vi "NF LI56xx sub init signal.vi"(7 "Type":string, 8 "error in":errorcluster caption="error in (no error)" {"code" format="%.0x"}, 11 "VISA resource name":refnum<visa-resource-name>) -> (0 "error out":errorcluster {"code" format="%.0x"}, 3 "VISA resource name copy":refnum<visa-resource-name>)   [LabVIEW 2019]
doc: "get input signal related parameters"
panel:
  in  "Measure Cluster":T1
  out "Measure Output Cluster":T2
  in  "Signal Cluster":T3
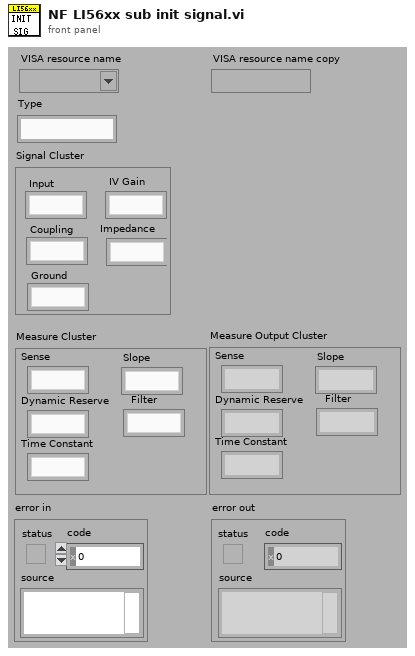
[diagram p1: front panel]
types:
  T1 = cluster{"Sense":string, "Dynamic Reserve":string, "Slope":string, "Filter":string, "Time Constant":string}
  T2 = cluster{"Sense":string, "Dynamic Reserve":string, "Time Constant":string, "Slope":string, "Filter":string}
  T3 = cluster{"Input":string, "Coupling":string, "Ground":string, "IV Gain":string, "Impedance":string}
  T4 = cluster{"input":string, "coupling":string, "ground":string, "IV gain":string, "impedance":string}
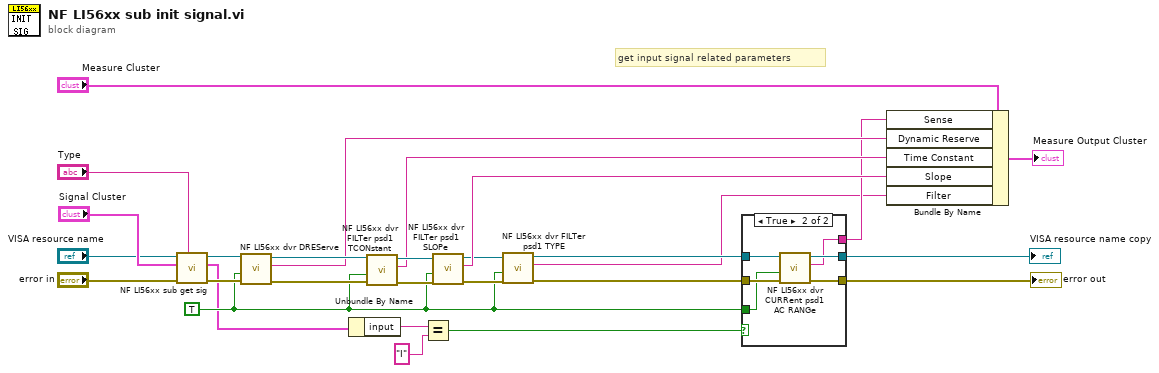
[diagram p0: block diagram]
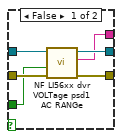
[diagram p2: hidden frame]
diagram:
  w3 = TRUE ("Read(F)")
  # "get input signal related parameters"
  n1 = call "NF LI56xx sub get sig.vi"("Type"="Type", "error in"="error in", "signal cluster"="Signal Cluster", "VISA resource name"="VISA resource name") -> ("error out"=w15:errorcluster, "output"=w2:T4, "VISA resource name copy"=w16:refnum<visa-resource-name>)  [unwired: 5 in]
  n2 = call "NF LI56xx dvr DREServe.vi"("error in"=w15, "Read(F)"=w3, "VISA resource name"=w16) -> ("error out"=w21:errorcluster, "query dynamic reserve"=w11:string, "VISA resource name copy"=w23:refnum<visa-resource-name>)  [unwired: 6 in]
  n3 = Unbundle By Name(w2) -> ("input"=w19:string)
  n4 = call "NF LI56xx dvr FILTer psd1 TCONstant.vi"("error in"=w21, "Read(F)"=w3, "VISA resource name"=w23) -> ("error out"=w20:errorcluster, "query time constnat"=w10:string, "VISA resource name copy"=w22:refnum<visa-resource-name>)  [unwired: 6 in]
  n5 = Equal?(x=w19, y="I" ("t")) -> (x = y?=w17:bool)
  n6 = call "NF LI56xx dvr FILTer psd1 SLOPe.vi"("error in"=w20, "Read(F)"=w3, "VISA resource name"=w22) -> ("error out"=w8:errorcluster, "query filter slope"=w12:string, "VISA resource name copy"=w6:refnum<visa-resource-name>)  [unwired: 6 in]
  n7 = call "NF LI56xx dvr FILTer psd1 TYPE.vi"("error in"=w8, "Read(F)"=w3, "VISA resource name"=w6) -> ("error out"=w7:errorcluster, "query filter slope"=w4:string, "VISA resource name copy"=w5:refnum<visa-resource-name>)  [unwired: 6 in]
  n8 = case shown="True" w17 {
    tunnel: w5 -> [w34 w40]
    tunnel: w7 -> [w33 w39]
    tunnel: [w32 w38] -> w14
    tunnel: [w31 w37] -> w13
    tunnel: [w30 w36] -> w9
    tunnel: w3 -> [w29 w35]
    frame False {
      n9 = call "NF LI56xx dvr VOLTage psd1 AC RANGe.vi"("error in"=w33, "Read(F)"=w29, "VISA resource name"=w34) -> ("error out"=w31:errorcluster, "query sensitivity"=w30:string, "VISA resource name copy"=w32:refnum<visa-resource-name>)  [unwired: 6 in]
    }
    frame True {
      n10 = call "NF LI56xx dvr CURRent psd1 AC RANGe.vi"("error in"=w39, "Read(F)"=w35, "VISA resource name"=w40) -> ("error out"=w37:errorcluster, "query sensitivity"=w36:string, "VISA resource name copy"=w38:refnum<visa-resource-name>)  [unwired: 6 in]
    }
  }
  "error out" <- w13
  "VISA resource name copy" <- w14
  n11 = Bundle By Name(cluster="Measure Cluster", "Sense"=w9, "Dynamic Reserve"=w11, "Time Constant"=w10, "Slope"=w12, "Filter"=w4) -> (→"Measure Output Cluster":T1)
